vi "createCommandList.vi"(8 "error in (no error)":errorcluster, 10 "Parameters":u32[](array[numeric]), 11 "HF-Felder in":refnum<class "HF-Felder.lvclass">) -> (0 "error out":errorcluster, 2 "Commandlist":string, 3 "HF-Felder out":refnum<class "HF-Felder.lvclass">)   [LabVIEW 2013, in "HF-Felder.lvclass"]
uses:
  HF-Felder.lvclass
panel:
  # "Modulation\n0 =  OFF\n1 = 2Hz\n2 = 400Hz\n3 = 1kHz\n4 = Pulse"
  # "dwelltime\n10 entspricht\n1sek"
  # "start Freq\nin kHz"
  # "stop Freq\nin kHz"
  # "Spannung\n10 entspricht 1V"
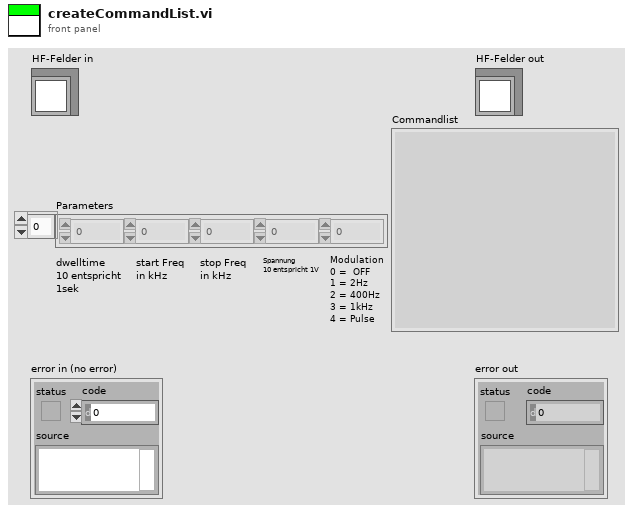
[diagram p1: front panel]
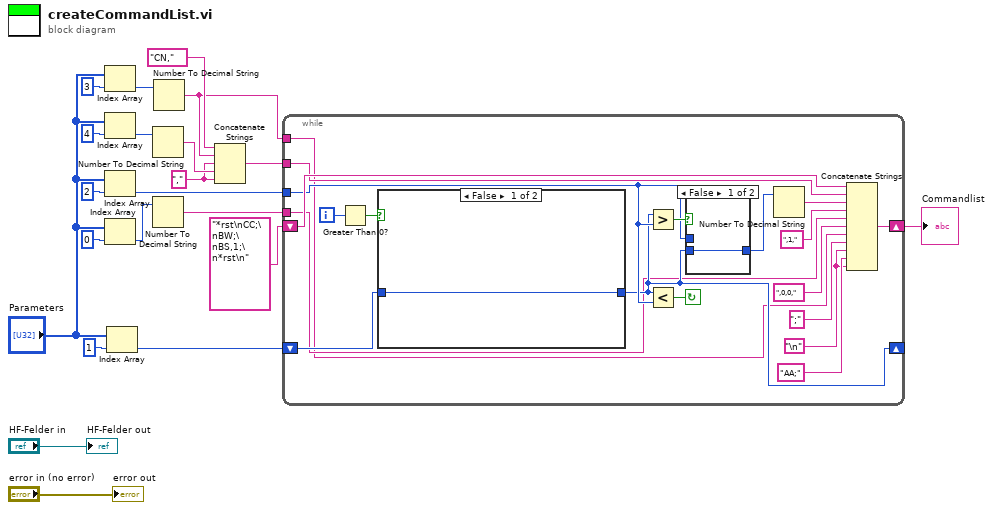
[diagram p0: block diagram]
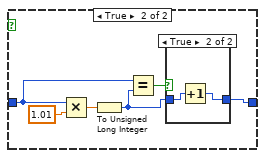
[diagram p2: hidden frame]
diagram:
  w1 = "," ("String")
  n1 = Index Array(array="Parameters", index=3) -> (element=w15:u32)
  n2 = Index Array(array="Parameters", index=4) -> (element=w3:u32)
  n3 = Index Array(array="Parameters", index=2) -> (element=w17:u32)
  n4 = Index Array(array="Parameters", index=0) -> (element=w8:u32)
  n5 = Index Array(array="Parameters", index=1) -> (element=w19:u32)
  n6 = Number To Decimal String(number=w3) -> (decimal integer string=w2:string)  [unwired: 1 in]
  n7 = Number To Decimal String(number=w8) -> (decimal integer string=w9:string)  [unwired: 1 in]
  n8 = Number To Decimal String(number=w15) -> (decimal integer string=w6:string)  [unwired: 1 in]
  n9 = Concatenate Strings("CN,", w6, w1, w2, w1) -> (w13:string)
  n10 = while {
    shift-right: [w40] -> w11
    shift-left: "*rst\nCC;\nBW;\nBS,1;\n*rst\n" -> [w39]
    tunnel: w13 -> [w38]
    tunnel: w17 -> [w33]
    shift-right: [w32] -> _
    shift-left: w19 -> [w35]
    tunnel: w9 -> [w28]
    tunnel: w6 -> [w22]
    i -> [w24]
    stop <- w36 continue-if-true
    w25 = "\n"
    n11 = Greater Than 0?(x=w24) -> (x > 0?=w23:bool)
    n12 = case shown="False" w23 {
      tunnel: w35 -> [w41 w45]
      tunnel: [w41 w44] -> w32
      frame False {
      }
      frame True {
        n13 = Multiply(x=w45, y=1.01) -> (x*y=w43:dbl)
        n14 = To Unsigned Long Integer(number=w43) -> (unsigned 32bit integer=w47:u32)
        n15 = Equal?(x=w45, y=w47) -> (x = y?=w46:bool)
        n16 = case shown="True" w46 {
          tunnel: w47 -> [w48 w49]
          tunnel: [w48 w50] -> w44
          frame False {
          }
          frame True {
            n17 = Increment(x=w49) -> (x+1=w50:u32)
          }
        }
      }
    }
    n18 = Greater?(x=w32, y=w33) -> (0:w34:bool)
    n19 = Less?(x=w32, y=w33) -> (x < y?=w36:bool)
    n20 = case shown="False" w34 {
      tunnel: w33 -> [_ w52]
      tunnel: w32 -> [w51 _]
      tunnel: [w51 w52] -> w31
      frame False {
      }
      frame True {
      }
    }
    n21 = Number To Decimal String(number=w31) -> (decimal integer string=w37:string)  [unwired: 1 in]
    n22 = Concatenate Strings(w39, w38, w37, ",1," ("string"), w28, ",0,0," ("string"), w22, ";" ("string"), w25, "AA;", w25) -> (w40:string)
  }
  "Commandlist" <- w11
  "error out" <- "error in (no error)"
  "HF-Felder out" <- "HF-Felder in"
